vi "Set LEDs.vi"() -> (3 "DSM Message":string)   [LabVIEW 2014, in "GEA2_Toolkit.lvlib"]
uses:
  Labview GEA2 Toolkit v2.1/library/GEA2_Toolkit.lvlib
  Custom Pallet Controls/Forward.ctl
panel:
  in  "G 5":bool
  in  "F 5":bool
  in  "E 5":bool
  in  "D 5":bool
  in  "C 5":bool
  in  "B 5":bool
  in  "A 5":bool
  in  "G 4":bool
  in  "F 4":bool
  in  "E 4":bool
  in  "D 4":bool
  in  "C 4":bool
  in  "B 4":bool
  in  "A 4":bool
  in  "G 3":bool
  in  "F 3":bool
  in  "E 3":bool
  in  "D 3":bool
  in  "C 3":bool
  in  "B 3":bool
  in  "A 3":bool
  in  "G 2":bool
  in  "F 2":bool
  in  "E 2":bool
  in  "D 2":bool
  in  "C 2":bool
  in  "B 2":bool
  in  "A 2":bool
  in  "G":bool
  in  "F":bool
  in  "E":bool
  in  "D":bool
  in  "C":bool
  in  "B":bool
  in  "A":bool
  out "Description":string="Set LEDs"
  in  "Complete":T1
  # "Discrete LED #2"
  # "Discrete LED #1"
  # "7-Segment Char#1"
  # "7-Segment Char#1"
  # "7-Segment Char#1"
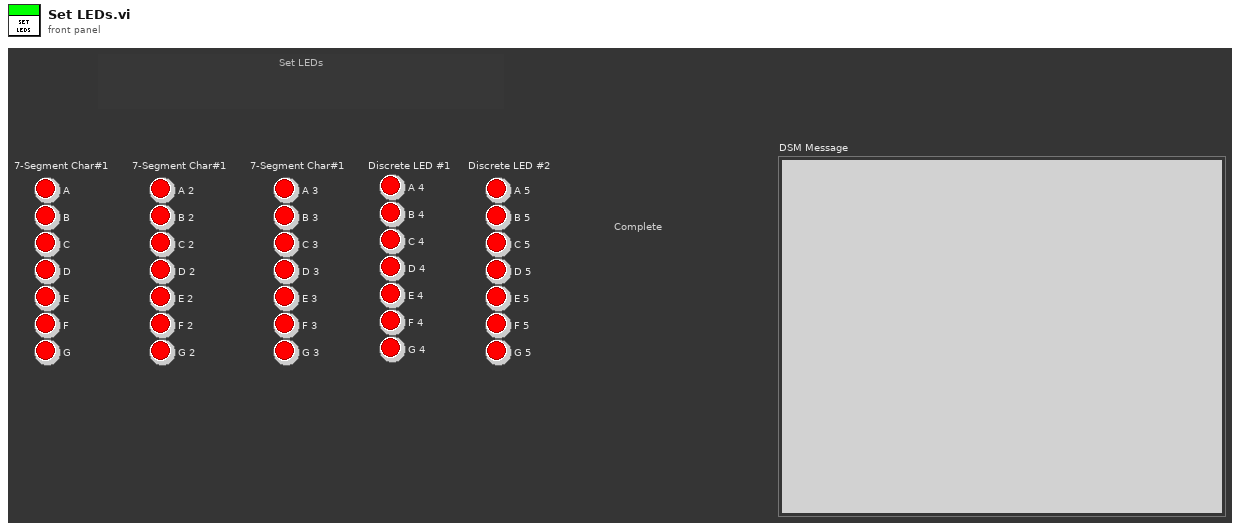
[diagram p1: front panel]
types:
  T1 = typedef "GEA2_Toolkit.lvlib/Forward.ctl" = bool
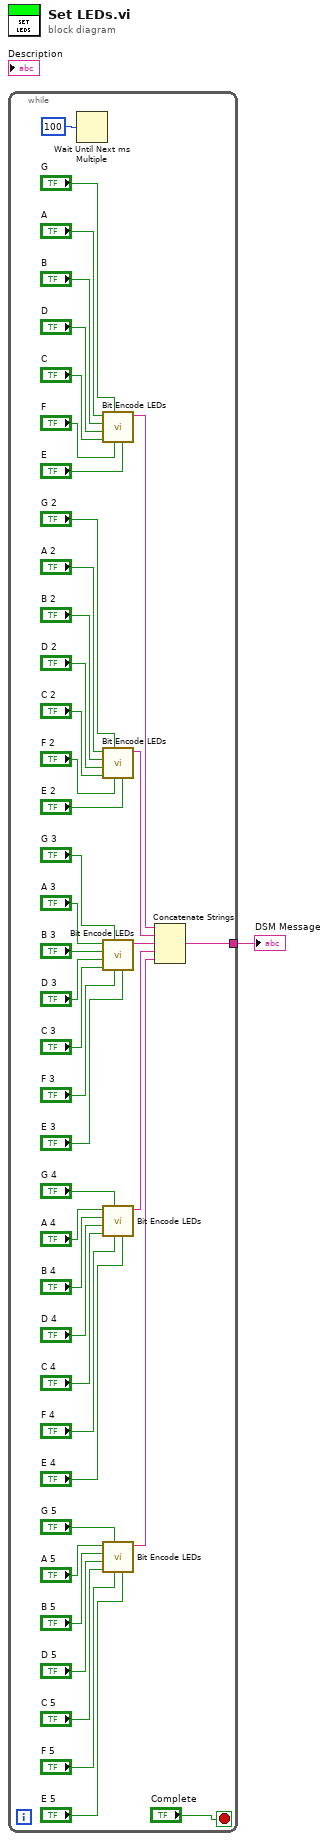
[diagram p0: block diagram]
diagram:
  n1 = while {
    tunnel: [w2] -> w1
    stop <- "Complete" stop-if-true
    n2 = Wait Until Next ms Multiple(millisecond multiple=u32 100) -> ()  [unwired: 1 out]
    n3 = call "Bit Encode LEDs.vi"("E"="E", "F"="F", "G"="G", "C"="C", "D"="D", "B"="B", "A"="A") -> ("String"=w7:string)  [unwired: 4 in]
    n4 = call "Bit Encode LEDs.vi"("E"="E 2", "F"="F 2", "G"="G 2", "C"="C 2", "D"="D 2", "B"="B 2", "A"="A 2") -> ("String"=w6:string)  [unwired: 4 in]
    n5 = call "Bit Encode LEDs.vi"("E"="E 3", "F"="F 3", "G"="G 3", "C"="C 3", "D"="D 3", "B"="B 3", "A"="A 3") -> ("String"=w5:string)  [unwired: 4 in]
    n6 = call "Bit Encode LEDs.vi"("E"="E 4", "F"="F 4", "G"="G 4", "C"="C 4", "D"="D 4", "B"="B 4", "A"="A 4") -> ("String"=w4:string)  [unwired: 4 in]
    n7 = call "Bit Encode LEDs.vi"("E"="E 5", "F"="F 5", "G"="G 5", "C"="C 5", "D"="D 5", "B"="B 5", "A"="A 5") -> ("String"=w3:string)  [unwired: 4 in]
    n8 = Concatenate Strings(w7, w6, w5, w4, w3) -> (w2:string)
  }
  "DSM Message" <- w1
